vi "Send Write Config Signal.vi"(7 "Message Priority (Normal)":T2=enum."Normal", 8 "error in (no error)":errorcluster, 10 "Config Signal":T1={"offset"=0.0, "square wave duty cycle (%)"=50.0, "reset signal"=FALSE, "sampling info"={"Fs"=1000.0, "#s"=1000.0}, "phase"=0.0, "signal type"=enum."Sine Wave", "amplitude"=1.0, "frequency"=10.0} {"frequency" format="%0.2p"; "amplitude" format="%0.2p"; "phase" format="%.2p"; "sampling info"."Fs" format="%.2p"; "square wave duty cycle (%)" format="%0.2f"; "offset" format="%0.2p"}, 11 "Message Enqueuer":refnum<class "Message Enqueuer.lvclass">) -> (0 "error out":errorcluster, 3 "Message Enqueuer out":refnum<class "Message Enqueuer.lvclass">)   [LabVIEW 2020, in "Generador.lvlib" / "Write Config Signal Msg.lvclass"]
doc: "This VI sends the message to an actor."
uses:
  Write Config Signal Msg.lvclass
  <vilib>/ActorFramework/Message Enqueuer/Message Enqueuer.lvclass
  <vilib>/ActorFramework/Message Enqueuer/Message Priority.ctl
  C:/Program Files (x86)/National Instruments/LabVIEW 2020/vi.lib/ActorFramework/Message/Message.lvclass
  Write Config Signal Msg.lvclass/Write Config Signal Msg.ctl
  <vilib>/ActorFramework/Message Enqueuer/Message Enqueuer.lvclass/Message Enqueuer.ctl
  <vilib>/ActorFramework/Message Priority Queue/Priority Enqueue.vi
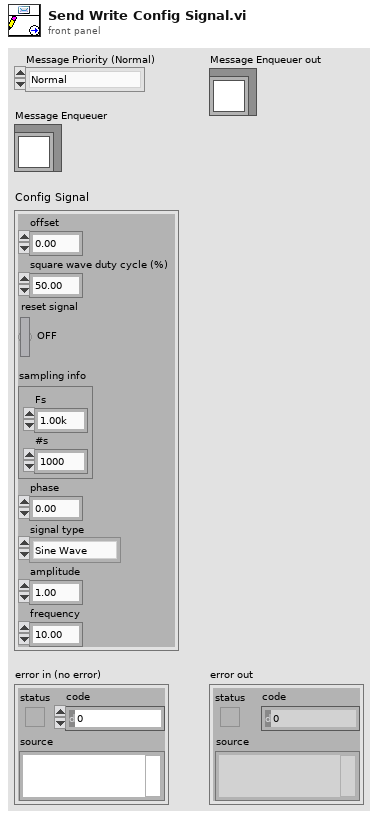
[diagram p1: front panel]
types:
  T1 = cluster{"offset":dbl, "square wave duty cycle (%)":dbl, "reset signal":bool, "sampling info":cluster{"Fs":dbl, "#s":dbl}, "phase":dbl, "signal type":enum16{"Sine Wave", "Triangle Wave", "Square Wave", "Sawtooth Wave"}, "amplitude":dbl, "frequency":dbl}
  T2 = typedef "Actor Framework.lvlib/Message Enqueuer.lvclass/Message Priority.ctl" = enum16{"Low", "Normal", "High"}
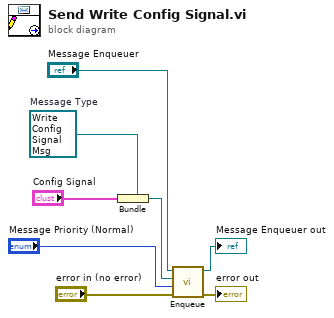
[diagram p0: block diagram]
diagram:
  w5 = refnum<class "Write Config Signal Msg.lvclass"> refnum  # Message Type
  n1 = Bundle(cluster=w5, "Config Signal") -> (w4:refnum<class "Write Config Signal Msg.lvclass">)
  n2 = call <vilib>:"Enqueue.vi"("error in (no error)"="error in (no error)", "Message Priority (Normal)"="Message Priority (Normal)", "Message"=w4, "Message Enqueuer in"="Message Enqueuer") -> ("error out"=→"error out":errorcluster, "Message Enqueuer out"=→"Message Enqueuer out":refnum<class "Message Enqueuer.lvclass">)  [unwired: 6 in]
